vi "Publish.vi"(8 "error in (no error)":errorcluster, 9 "Payload":string, 10 "Topic":string, 11 "MQTT1 in":refnum<class "MQTT1.lvclass">) -> (0 "error out":errorcluster, 3 "MQTT1 out":refnum<class "MQTT1.lvclass">)   [LabVIEW 2017, in "MQTT1.lvclass"]
uses:
  MQTT1.lvclass
  Libraries/mqtt Folder/src/class/mqtt/mqtt.lvclass
panel:
  out "success":bool
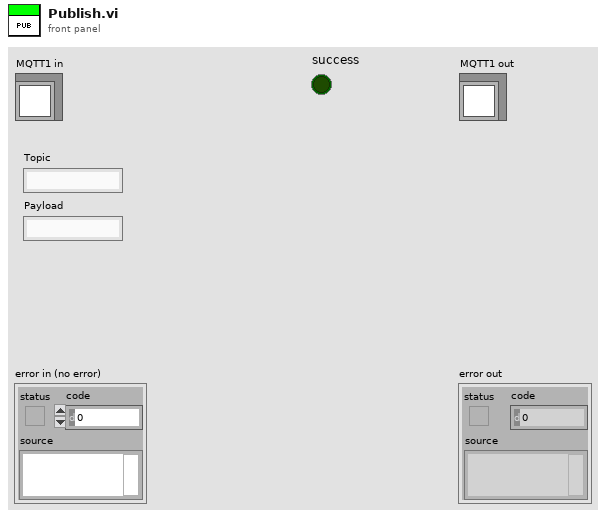
[diagram p1: front panel]
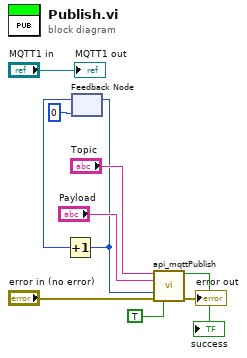
[diagram p0: block diagram]
diagram:
  n1 = feedback #1(u16 0) -> (w6:u16)
  n2 = Increment(x=w6) -> (x+1=w5:u16)
  n3 = feedback-in #1(w5) -> ()
  n4 = call "api_mqttPublish.vi"("topic"="Topic", "value"="Payload", "messageID"=w5, "error in (no error)"="error in (no error)", "retain(F)"=TRUE) -> ("success"=→"success":bool, "error out"=→"error out":errorcluster)  [unwired: 9 in]
  "MQTT1 out" <- "MQTT1 in"
